vi "Get Error in from Terminals Info.vi"(11 "terminals info":T1) -> (2 "error in terms indexes":i32[](array[numeric]), 3 "error wires inside refs[]":refnum<vi>[](array[refnum]))   [LabVIEW 2014]
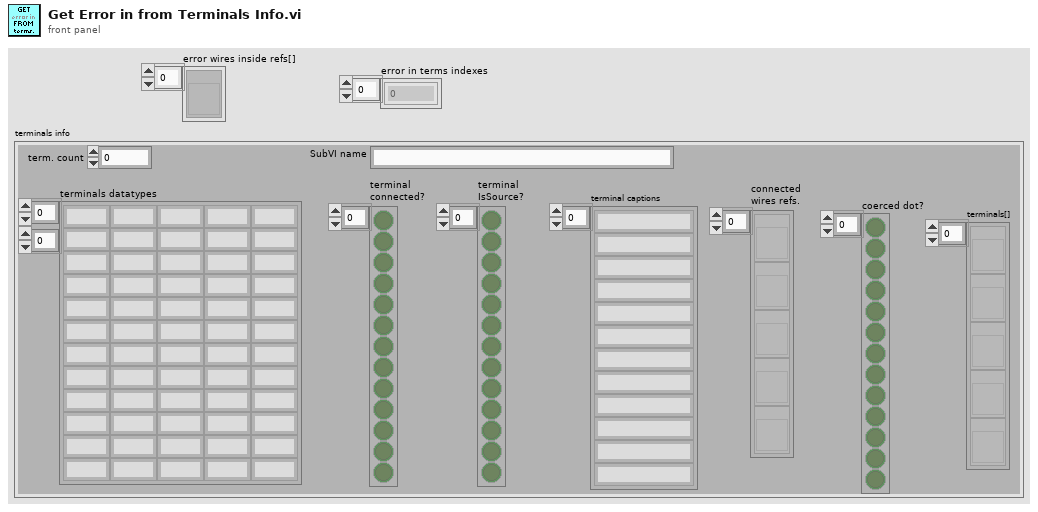
[diagram p1: front panel]
types:
  T1 = cluster{"terminals datatypes":string[][], "terminal\nconnected?":bool[], "terminal captions":string[], "term. count":i32, "terminal\nIsSource?":bool[], "SubVI name":string, "connected\nwires refs.":refnum<vi>[], "coerced dot?":bool[], "terminals[]":refnum<vi>[]}
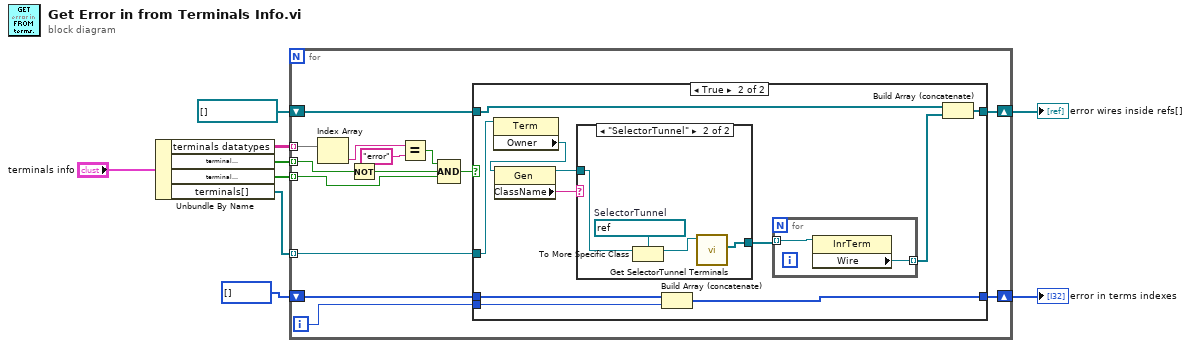
[diagram p0: block diagram]
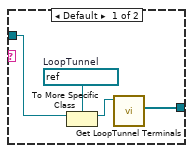
[diagram p3: hidden frame]
diagram:
  n1 = Unbundle By Name("terminals info") -> ("terminals datatypes"=w9:string[][], "terminal\nIsSource?"=w8:bool[], "terminal\nconnected?"=w6:bool[], "terminals[]"=w3:refnum<vi>[])
  n2 = for {
    tunnel: w9 -> [w23] mode=indexing
    tunnel: w8 -> [w19] mode=indexing
    shift-right: [w16] -> w5
    shift-left: refnum<vi>[] [] ("connected\nwires refs.") -> [w17]
    tunnel: w6 -> [w15] mode=indexing
    tunnel: w3 -> [w13] mode=indexing
    shift-right: [w11] -> w1
    shift-left: i32[] [] -> [w12]
    i -> [w10]
    n3 = Index Array(array=w23) -> (element=w22:string)  [unwired: 1 in]
    n4 = Not(x=w19) -> (.not. x?=w14:bool)
    n5 = Equal?(x=w22, y="error") -> (x = y?=w20:bool)
    n6 = Compound Arithmetic op=AND(w20, w14, w15) -> (w18:bool)
    n7 = case shown="True" w18 {
      tunnel: [w25 w35] -> w16
      tunnel: w17 -> [w25 w36]
      tunnel: w13 -> [_ w27]
      tunnel: w12 -> [w24 w34]
      tunnel: [w24 w33] -> w11
      tunnel: w10 -> [_ w32]
      frame False {
      }
      frame True {
        n8 = property class="Term"(reference=w27) -> ("Owner"=w29:refnum<vi>)  [unwired: 1 in, 2 out]
        n9 = property class="Gen"(reference=w29) -> (reference out=w26:refnum<vi>, "ClassName"=w28:string)  [unwired: 1 in, 1 out]
        n10 = case shown="\"SelectorTunnel\"" w28 {
          tunnel: [w40 w44] -> w30
          tunnel: w26 -> [w37 w41]
          frame Default {
            w38 = refnum<vi> refnum  # LoopTunnel
            n11 = To More Specific Class(target class=w38, reference=w37) -> (specific class reference=w39:refnum<vi>)  [unwired: 1 in, 1 out]
            n12 = call "Get LoopTunnel Terminals.vi"("LoopTunnel in"=w39) -> ("Inside Terminals[]"=w40:refnum<vi>[])  [unwired: 7 in, 3 out]
          }
          frame "SelectorTunnel" {
            w43 = refnum<vi> refnum  # SelectorTunnel
            n13 = To More Specific Class(target class=w43, reference=w41) -> (specific class reference=w42:refnum<vi>)  [unwired: 1 in, 1 out]
            n14 = call "Get SelectorTunnel Terminals.vi"("SelectorTunnel in"=w42) -> ("Inside Terminals[]"=w44:refnum<vi>[])  [unwired: 7 in, 3 out]
          }
        }
        n15 = Build Array (concatenate)(w34, w32) -> (w33:i32[])
        n16 = for {
          tunnel: [w46] -> w31 mode=indexing
          tunnel: w30 -> [w45] mode=indexing
          n17 = property class="InrTerm"(reference=w45) -> ("Wire"=w46:refnum<vi>)  [unwired: 1 in, 2 out]
        }
        n18 = Build Array (concatenate)(w36, w31) -> (w35:refnum<vi>[])
      }
    }
  }
  "error wires inside refs[]" <- w5
  "error in terms indexes" <- w1
